vi "Query Platform System Time.vi"(0 "VISA resource name":refnum<visa-resource-name>, 11 "error in (no error)":errorcluster) -> (4 "VISA resource name out":refnum<visa-resource-name>, 6 "Hour":i16, 8 "Minute":i16, 10 "Second":i16, 15 "error out":errorcluster)   [LabVIEW 2018, in "LTB-1.lvlib" / "3150.lvlib"]
doc: "The device has an internal clock and implements the SYSTem:TIME command to get the clock time over the interface."
uses:
  3150.lvlib
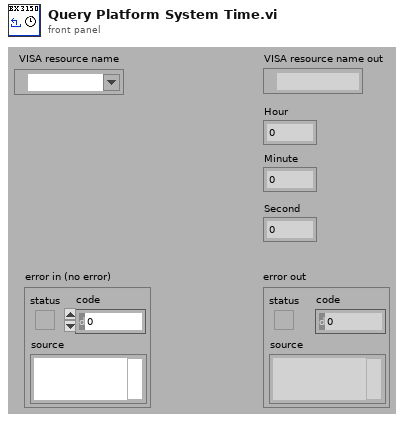
[diagram p1: front panel]
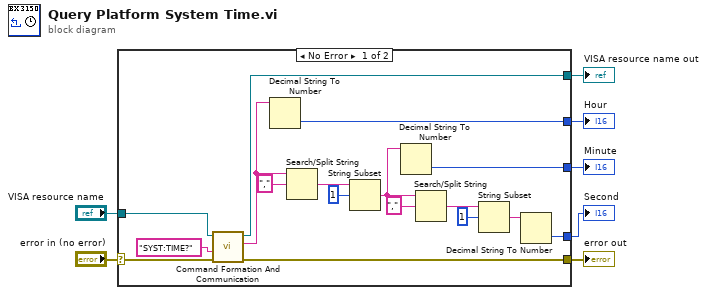
[diagram p0: block diagram]
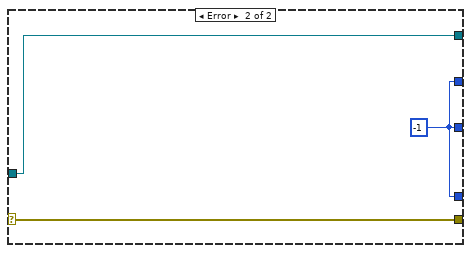
[diagram p2: hidden frame]
diagram:
  n1 = case shown="No Error" "error in (no error)" {
    selector: "error in (no error)" -> [w13 w27]
    tunnel: [w12 w26] -> w6
    tunnel: [w11 w27] -> w4
    tunnel: [w17 w25] -> w1
    tunnel: [w16 w25] -> w3
    tunnel: [w15 w25] -> w2
    tunnel: "VISA resource name" -> [w8 w26]
    frame No Error {
      n2 = call "Command Formation And Communication.vi"("error in (no error)"=w13, "Command"="SYST:TIME?", "VISA resource name"=w8) -> ("error out"=w11:errorcluster, "Response"=w10:string, "VISA resource name out"=w12:refnum<visa-resource-name>)  [unwired: 1 in, 5 out]
      n3 = Decimal String To Number(string=w10) -> (number=w17:i32)  [unwired: 3 out]
      n4 = Search/Split String(string=w10, search string/char (-)=",") -> (match + rest of string=w23:string)  [unwired: 3 out]
      n5 = String Subset(string=w23, offset (0)=1) -> (substring=w21:string)  [unwired: 1 out]
      n6 = Decimal String To Number(string=w21) -> (number=w16:i32)  [unwired: 3 out]
      n7 = Search/Split String(string=w21, search string/char (-)=",") -> (match + rest of string=w19:string)  [unwired: 3 out]
      n8 = String Subset(string=w19, offset (0)=1) -> (substring=w18:string)  [unwired: 1 out]
      n9 = Decimal String To Number(string=w18) -> (number=w15:i32)  [unwired: 3 out]
    }
    frame Error {
      w25 = -1
    }
  }
  "VISA resource name out" <- w6
  "error out" <- w4
  "Hour" <- w1
  "Second" <- w2
  "Minute" <- w3
